vi "Save.vi"(7 "source paths":path[](array[path]), 8 "error in (no error)":errorcluster, 10 "processed sources":refnum<class "AB_Source.lvclass">[](array[class]), 11 "AB_DLL in":refnum<class "AB_DLL.lvclass">) -> (0 "error out":errorcluster, 1 "TypeInfo":string, 2 "source destination paths":path[](array[path]), 3 "AB_DLL out":refnum<class "AB_DLL.lvclass">, 4 "LEIFBuildData":u32, 5 "checksums":string[](array[string]))   [LabVIEW 2020, in "AB_DLL.lvclass"]
uses:
  <vilib>/AppBuilder/AB_Classes/DLL/AB_DLL.lvclass
  e:/builds/penguin/labview/branches/2020/dev/dist/vi.lib/AppBuilder/AB_Classes/TargetFile/AB_Targetfile.lvclass
  <vilib>/AppBuilder/AB_Classes/Source/AB_Source.lvclass
  <vilib>/AppBuilder/AB_Classes/Application/AB_Application.lvclass
  <vilib>/AppBuilder/AB_Classes/TargetFile/AB_Targetfile.lvclass
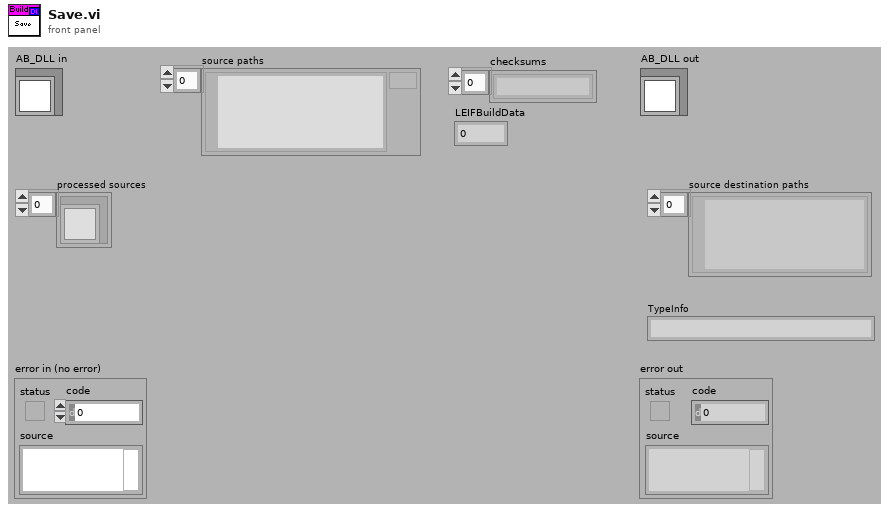
[diagram p1: front panel]
types:
  T1 = typedef "AB_Targetfile.ctl" = cluster{"targetfileName":string, "targetfileGUID":string, "enableDebugging":bool, "versionInfo":cluster{"productName":string, "legalCopyright":string, "companyName":string, "internalName":string, "fileDescription":string}, "eng_consolidatedTypeInfo":string, "fastFileFormat":bool, "eng_LEIFBuildData":u32, "versionIndependent":bool}
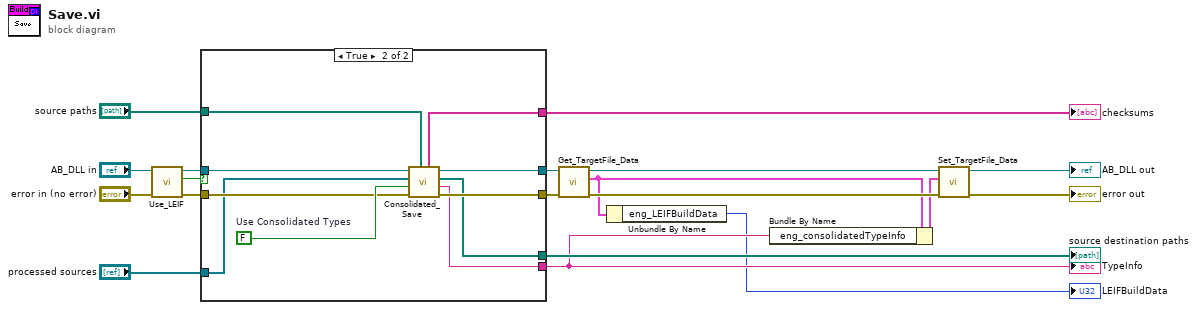
[diagram p0: block diagram]
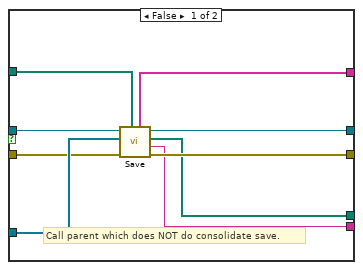
[diagram p2: hidden frame]
diagram:
  n1 = call <vilib>:"Use_LEIF.vi"("error in (no error)"="error in (no error)", "AB_Targetfile in"="AB_DLL in") -> ("error out"=w4:errorcluster, "use LEIF?"=w1:bool, "AB_Targetfile out"=w2:refnum<class "AB_DLL.lvclass">)  [unwired: 7 in]
  n2 = case shown="True" w1 {
    tunnel: "processed sources" -> [w24 w31]
    tunnel: w4 -> [w23 w34]
    tunnel: [w27 w35] -> w9
    tunnel: [w28 w36] -> w11
    tunnel: [w20 w29] -> w8
    tunnel: "source paths" -> [w22 w33]
    tunnel: [w26 w30] -> w17
    tunnel: w2 -> [w25 w37]
    tunnel: [w21 w32] -> w16
    frame False {
      # "Call parent which does NOT do consolidate save."
      n3 = call-parent "Save.vi"("source paths"=w22, "error in"=w23, "processed sources"=w24, "AB_Build in"=w25) -> ("error out"=w27:errorcluster, "TypeInfo"=w20:string, "source destination paths"=w26:path[], "AB_Build out"=w28:refnum<class "AB_DLL.lvclass">, "checksums"=w21:string[])  [unwired: 2 in, 1 out]
    }
    frame True {
      w38 = FALSE  # Use Consolidated Types
      n4 = call <vilib>:"Consolidated_Save.vi"("source paths"=w33, "error in"=w34, "Use Consolidated Types"=w38, "processed sources"=w31, "AB_Targetfile in"=w37) -> ("error out"=w35:errorcluster, "TypeInfo"=w29:string, "source destination paths"=w30:path[], "AB_Targetfile out"=w36:refnum<class "AB_DLL.lvclass">, "checksums"=w32:string[])  [unwired: 2 in]
    }
  }
  "source destination paths" <- w17
  "TypeInfo" <- w8
  "checksums" <- w16
  n5 = call <vilib>:"Get_TargetFile_Data.vi"("error in (no error)"=w9, "AB_Targetfile in"=w11) -> ("error out"=w14:errorcluster, "data"=w7:T1, "AB_Targetfile out"=w15:refnum<class "AB_DLL.lvclass">)  [unwired: 7 in]
  n6 = Unbundle By Name(w7) -> ("eng_LEIFBuildData"=→"LEIFBuildData":u32)
  n7 = Bundle By Name(cluster=w7, "eng_consolidatedTypeInfo"=w8) -> (w13:T1)
  n8 = call <vilib>:"Set_TargetFile_Data.vi"("error in (no error)"=w14, "data"=w13, "AB_Targetfile in"=w15) -> ("error out"=→"error out":errorcluster, "AB_Targetfile out"=→"AB_DLL out":refnum<class "AB_DLL.lvclass">)  [unwired: 7 in]
